vi "Query Wavelength.vi"(8 "error in (no error)":errorcluster, 11 "VISA resource name":refnum<visa-resource-name>) -> (0 "error out":errorcluster, 2 "CURRENT WAVELENGTH":dbl[unit] min=0.0 max=0.0001677721500000001 step=1.0000000000000007e-09 format="%.2f", 3 "VISA resource name out":refnum<visa-resource-name>)   [LabVIEW 2017, in "Digikrom DK24x.lvlib"]
doc: "Returns the current wavelength setting."
uses:
  Digikrom DK24x.lvlib
  Private/Command.ctl
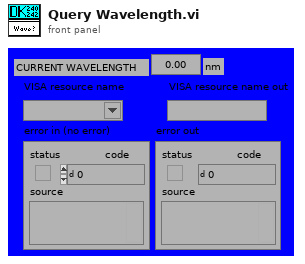
[diagram p1: front panel]
types:
  T1 = typedef "Digikrom DK24x.lvlib/Command.ctl" = u8
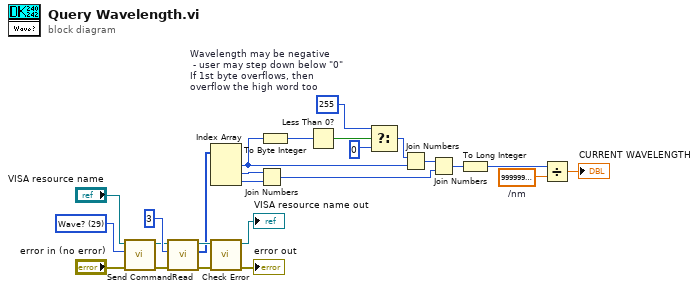
[diagram p0: block diagram]
diagram:
  w1 = T1 29 items=["Cancel"=24, "Clear"=25, "CSR"=28, "Echo"=27, "Filter"=15, "Gcal"=18, "Goto"=16, "Grtid?"=19, "Grtsel"=26, "NOVRAM Read"=56, "NOVRAM Write"=59, "Reset"=255, "Scan"=12, "Scan Up"=9, "Scan Down"=3, "Serial?"=33, "Slew Up"=8, "Slew Down"=2, "Slit Reset"=43, "Slit?"=30, "Sltadj"=14, "Speed"=13, "Sspeed?"=21, "Step Down"=1, "Step Up"=7, "S1adj"=31, "S2adj"=32, "S3adj"=34, "S1cal"=22, "S2cal"=23, "S3cal"=35, "Test"=17, "Type"=57, "Wave?"=29, "Zero"=52] ("Command")
  w6 = u8 255  # Wavelength may be negative  - user may step down below "0" If 1st byte overflows, then  overflow the high word too
  w23 = dbl[unit] 99999999999.99994  # /nm
  n1 = call "Send Command.vi"("error in (no error)"="error in (no error)", "Command"=w1, "VISA resource name"="VISA resource name") -> ("error out"=w10:errorcluster, "VISA resource name out"=w11:refnum<visa-resource-name>)  [unwired: 7 out]
  n2 = call "Read.vi"("error in (no error)"=w10, "response size"=u8 3, "VISA resource name"=w11) -> ("error out"=w20:errorcluster, "response array"=w14:u8[], "VISA resource name out"=w21:refnum<visa-resource-name>)  [unwired: 6 out]
  n3 = Index Array(array=w14) -> (element #1=w4:u8, element #2=w13:u8, element #3=w12:u8)  [unwired: 3 in]
  n4 = call "Check Error.vi"("error in"=w20, "VISA resource name in"=w21) -> ("error out"=→"error out":errorcluster, "VISA resource name out"=→"VISA resource name out":refnum<visa-resource-name>)  [unwired: 1 in, 7 out]
  n5 = Join Numbers(hi=w13, lo=w12) -> ((hi.lo)=w25:u16)
  n6 = To Byte Integer(number=w4) -> (8bit integer=w9:i8)
  n7 = Less Than 0?(x=w9) -> (x < 0?=w8:bool)
  n8 = Select(t=w6, s=w8, f=u8 0) -> (s? t:f=w3:u8)
  n9 = Join Numbers(hi=w3, lo=w4) -> ((hi.lo)=w2:u16)
  n10 = Join Numbers(hi=w2, lo=w25) -> ((hi.lo)=w24:u32)
  n11 = To Long Integer(number=w24) -> (32bit integer=w7:i32)
  n12 = Divide(x=w7, y=w23) -> (x/y=→"CURRENT WAVELENGTH":dbl[unit])
